vi "Read Str.vi"(8 "Error In":errorcluster, 11 "Reader In":refnum<class "Reader.lvclass">) -> (0 "Error Out":errorcluster, 2 "Value":string, 3 "Reader Out":refnum<class "Reader.lvclass">)   [LabVIEW 2019, in "LabPack.lvlib" / "Reader.lvclass"]
doc: "Reads and decodes a string from the MessagePack data."
uses:
  Reader.lvclass
  Reader.lvclass/Reader.ctl
  Private/Read Bytes by Value.vi
  Private/Handle Error.vi
  Status/Read Status.vi
  Status/Read Status Message.vi
  Status/Read Is Error.vi
  Private/Begin Str by Value.vi
  Utility/Status Code.vi
  <vilib>/Utility/error.llb/Error Cluster From Error Code.vi
  Private/End Str by Value.vi
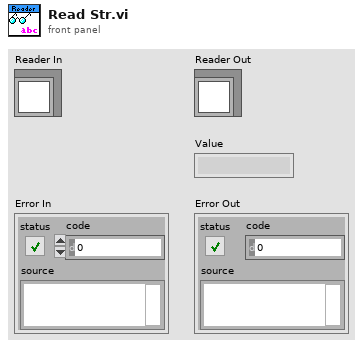
[diagram p1: front panel]
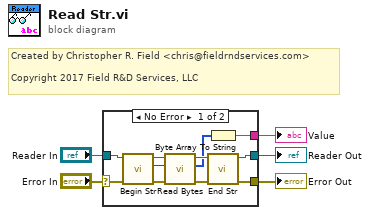
[diagram p0: block diagram]
diagram:
  # "Created by Christopher R. Field <chris@fieldrndservices.com>\n\nCopyright 2017 Field R&D Services, LLC"
  n1 = case shown="No Error" "Error In" {
    selector: "Error In" -> [w15 w17]
    tunnel: "Reader In" -> [w16 w18]
    tunnel: [w13 w17] -> w3
    tunnel: [w14 w18] -> w2
    tunnel: [w6 _] -> w1
    frame No Error {
      n2 = call-poly "Begin Str.vi"("Error In"=w15, "Reader In"=w16) -> ("Error Out"=w11:errorcluster, "Length"=w10:u32, "Reader Out"=w12:refnum<class "Reader.lvclass">)  [unwired: 7 in]
      n3 = call-poly "Read Bytes.vi"("Error In"=w11, "Count"=w10, "Reader In"=w12) -> ("Error Out"=w8:errorcluster, "Bytes"=w7:u8[], "Reader Out"=w9:refnum<class "Reader.lvclass">)  [unwired: 6 in]
      n4 = Byte Array To String(unsigned byte array=w7) -> (string=w6:string)
      n5 = call-poly "End Str.vi"("Error In"=w8, "Reader In"=w9) -> ("Error Out"=w13:errorcluster, "Reader Out"=w14:refnum<class "Reader.lvclass">)  [unwired: 8 in]
    }
    frame Error {
    }
  }
  "Error Out" <- w3
  "Reader Out" <- w2
  "Value" <- w1
